vi "Run Test Suite.vi"(8 "error in (no error)":errorcluster, 10 "Test Case":refnum<class "LUnit Test Suite.lvclass">, 11 "Execution API In":refnum<class "Execution API.lvclass">) -> (0 "error out":errorcluster, 3 "Execution API Out":refnum<class "Execution API.lvclass">)   [LabVIEW 2020, in "Execution API.lvclass"]
uses:
  Execution API.lvclass
  C:/Users/anton/Documents/GitHub/LUnit/source/Application Framework/Process Classes/Process/Process.lvclass
  Test Suite/LUnit Test Suite.lvclass
  Application Framework/Process Classes/Process/Process.lvclass/Process.ctl
  Application Framework/Process Classes/Process/Process.lvclass
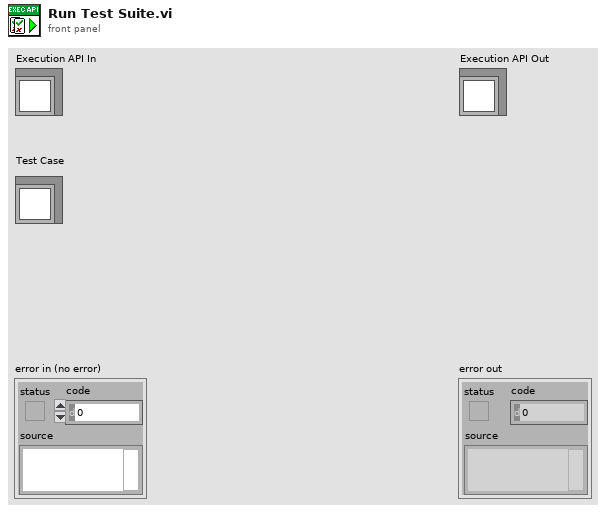
[diagram p1: front panel]
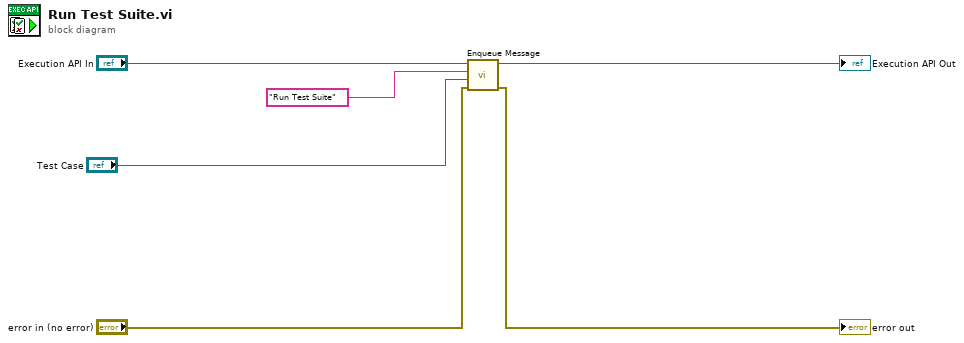
[diagram p0: block diagram]
diagram:
  n1 = call "Enqueue Message.vi"("error in (no error)"="error in (no error)", "Message Data"="Test Case", "Message"="Run Test Suite", "Process In"="Execution API In") -> ("error out"=→"error out":errorcluster, "Process Out"=→"Execution API Out":refnum<class "Execution API.lvclass">)  [unwired: 6 in]
